vi "GageTransfer-LowOverheadMod.vi"(0 "Handle Cluster":T1, 1 "Start (0)":dbl, 2 "Length (4096)":dbl=4096.0, 5 "Buffer in I32":i32[](array[numeric]), 7 "Buffer in I16":i16[](array[numeric]), 9 "Buffer in U8":u8[](array[numeric]), 12 "Channel (0)":u16 step=1, 13 "Mode (0)":u32 step=1, 14 "Segment (1)":u32=1) -> (3 "Actual Length":dbl, 4 "Actual Start":dbl, 6 "Buffer Out I32":i32[](array[numeric]), 8 "Buffer Out I16":i16[](array[numeric]), 10 "Buffer Out U8":u8[](array[numeric]), 15 "Error Code":i32)   [LabVIEW 2014, in "GageLv.lvlib"]
doc: "This VI transfers the data from one channel of the CompuScope system identified by Handle Cluster, which is obtained by calling CsTool-GetSystem.vi. For accurate interpretation of the transferred data, the user should always use the returned Actual Start and Actual Length, and not the requested values. \n\nThis VI can be used for transferring data from 8, 12, 14, and 16 bit CompuScope hardware. Data are transferred from on-board CompuScope memory to PC RAM using PCI Bus Mastering at rates of up to 200 MB/s. \n\nInternally, CsTool-Transfer.vi converts the raw integer ADC code values into double variable voltage values. For more rapid data access, the user may remove the voltage conversion step. The VI will not return programmatic control to LabVIEW until all of the data have been transferred. \n\nIf the call is successful, a 1 is returned in the Error Code indicator. If the call is unsuccessful, an appropriate error code is returned. A descriptive error string may be obtained by calling CsTool-ErrorHandler.vi.\n\n\nInput Value Descriptions:\n\nChannel\nThis integer value specifies the channel from which data are to be transferred. The default value is 0 for the first channel in the CompuScope system. Channels in a LabVIEW CompuScope system begin at 0. If an invalid channel number is given, an error will be returned. Please see the CompuScope hardware manual for more information on channel enumeration.\n\nMode\nThis integer value determines the current transfer mode. Currently, the only valid value for this input is 0.\n\nSegment(1)\nThis integer value determines which Multiple Record segment is to be transferred, if the CompuScope hardware was operating in Multiple Record Mode. For Single Record Mode acquisitions, the user must always set the Record value to 1, which is the default value. If the Record value is too large, an error code will be returned. \n\nStart\nThis double variable value determines the requested starting point of the data transfer from CompuScope memory to PC RAM. Start is specified relative to the trigger address for the acquisition. A Start value of 0 will cause data transfer to begin at the trigger address. Negative Start values are used for the transfer of pre-trigger data. Positive Start values may be used to begin transfer after the trigger address. The default Start value is 0. \n\nLength\nThis double variable value specifies the amount of data, in samples, to be transferred. The default value is 4096. \n\nData in Volts\nThis array variable, of type double, is the LabVIEW buffer variable into which transferred data are returned. The size of the array will be at least Length samples. Data are returned as voltage values, whose conversion depends upon the resolution of the CompuScope system and on the current input range.\n\nActual Start\nThis double variable value returns the actual start point of the data array. The Actual Start may be lower than the requested Start value. This is because the CompuScope memory architecture may force the drivers to download data from an earlier point than the start position. For example, if Start is input to CsTool-Transfer.vi as 0, the Actual Start may return as -2, indicating that two extra samples were returned before the Start position. \n\nThe user must account for the discrepancy between the Start and the Actual Start. The user may choose to ignore samples transferred from before the Start position. Alternatively, the user may conserve these samples, accounting for the fact that the values begin at Actual Start. \n\nActual Length\nThis double variable value returns the actual amount of data transferred, which may be different from the requested Length. The difference, if any, results from CompuScope memory architecture."
uses:
  <instrlib>/GageLv_uic/GageLv.lvlib
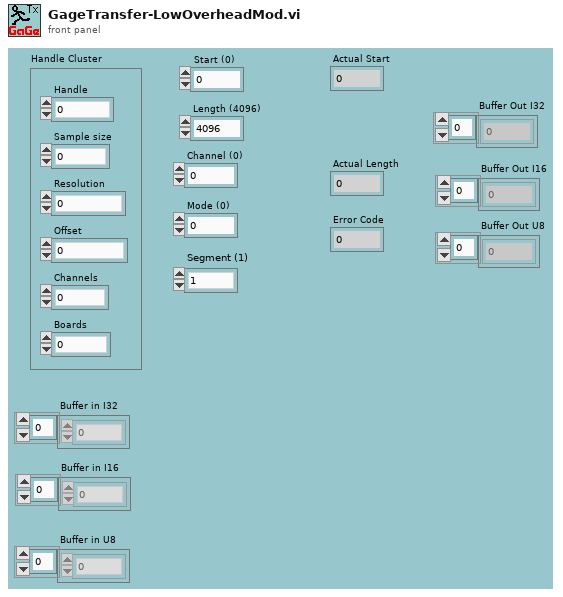
[diagram p1: front panel]
types:
  T1 = cluster{"Handle":u32, "Sample size":u32, "Resolution":i32, "Offset":i32, "Channels":u32, "Boards":u32}
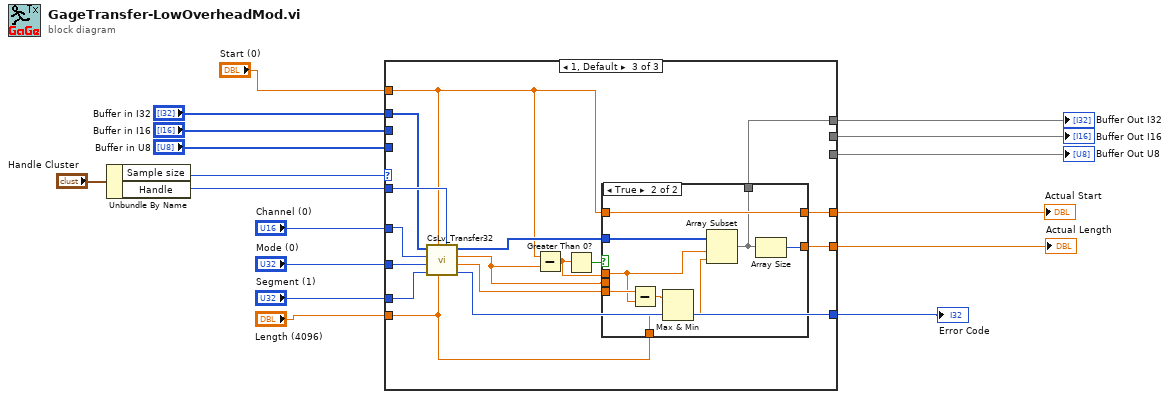
[diagram p0: block diagram]
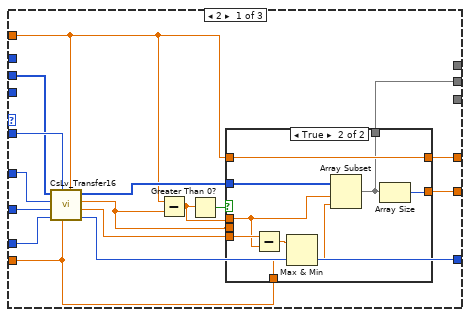
[diagram p2: hidden frame]
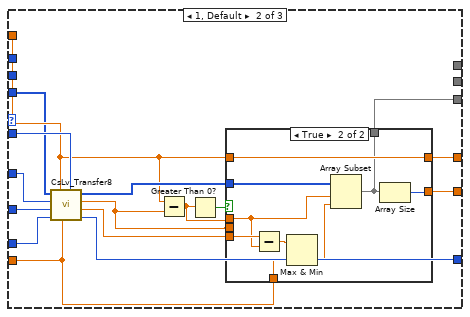
[diagram p4: hidden frame]
diagram:
  n1 = Unbundle By Name("Handle Cluster") -> ("Sample size"=w17:u32, "Handle"=w16:u32)
  n2 = case shown="1, Default" w17 {
    tunnel: "Length (4096)" -> [w24 w52 w80]
    tunnel: "Segment (1)" -> [w31 w59 w87]
    tunnel: "Mode (0)" -> [w30 w58 w86]
    tunnel: "Start (0)" -> [w23 w51 w79]
    tunnel: [w33 w61 w89] -> w13
    tunnel: w16 -> [w32 w60 w88]
    tunnel: "Channel (0)" -> [w29 w57 w85]
    tunnel: "Buffer in U8" -> [_ w48 _]
    tunnel: "Buffer in I16" -> [w18 _ _]
    tunnel: "Buffer in I32" -> [_ _ w74]
    tunnel: [w22 w50 w78] -> w6
    tunnel: [w21 w49 w77] -> w5
    tunnel: [w20 _ _] -> w4
    tunnel: [_ w47 _] -> w2
    tunnel: [_ _ w76] -> w1
    frame 2 {
      n3 = call <instrlib>:"CsLv_Transfer16.vi"("Start (0)"=w23, "Length (4096)"=w24, "Handle"=w32, "Segment (1)"=w31, "Mode (0)"=w30, "Channel (0)"=w29, "Buffer in I16"=w18) -> ("Error Code"=w33:i32, "Actual Length"=w25:dbl, "Actual Start"=w19:dbl, "Buffer"=w26:i16[])  [unwired: 1 in]
      n4 = Subtract(x=w23, y=w19) -> (x-y=w28:dbl)
      n5 = Greater Than 0?(x=w28) -> (x > 0?=w27:bool)
      n6 = case shown="True" w27 {
        tunnel: w28 -> [_ w43]
        tunnel: w25 -> [w36 w44]
        tunnel: [w36 w45] -> w22
        tunnel: w24 -> [_ w40]
        tunnel: w26 -> [w34 w39]
        tunnel: [w35 w38] -> w21
        tunnel: w23 -> [_ w38]
        tunnel: w19 -> [w35 _]
        tunnel: [w34 w37] -> w20
        frame False {
        }
        frame True {
          n7 = Subtract(x=w44, y=w43) -> (x-y=w42:dbl)
          n8 = Max & Min(x=w42, y=w40) -> (min(x,y)=w41:dbl)  [unwired: 1 out]
          n9 = Array Subset(array=w39, index=w43, length=w41) -> (w37:i16[])
          n10 = Array Size(array=w37) -> (size(s)=w45:i32)
        }
      }
    }
    frame 1, Default {
      n11 = call <instrlib>:"CsLv_Transfer8.vi"("Handle"=w60, "Length (4096)"=w52, "Start (0)"=w51, "Segment (1)"=w59, "Mode (0)"=w58, "Channel (0)"=w57, "Buffer in"=w48) -> ("Error Code"=w61:i32, "Actual Length"=w53:dbl, "Actual Start"=w46:dbl, "Buffer out"=w54:u8[])  [unwired: 1 in]
      n12 = Subtract(x=w51, y=w46) -> (x-y=w56:dbl)
      n13 = Greater Than 0?(x=w56) -> (x > 0?=w55:bool)
      n14 = case shown="True" w55 {
        tunnel: w56 -> [_ w71]
        tunnel: w53 -> [w64 w72]
        tunnel: [w64 w73] -> w50
        tunnel: w52 -> [_ w68]
        tunnel: w54 -> [w62 w67]
        tunnel: [w63 w66] -> w49
        tunnel: w51 -> [_ w66]
        tunnel: w46 -> [w63 _]
        tunnel: [w62 w65] -> w47
        frame False {
        }
        frame True {
          n15 = Subtract(x=w72, y=w71) -> (x-y=w70:dbl)
          n16 = Max & Min(x=w70, y=w68) -> (min(x,y)=w69:dbl)  [unwired: 1 out]
          n17 = Array Subset(array=w67, index=w71, length=w69) -> (w65:u8[])
          n18 = Array Size(array=w65) -> (size(s)=w73:i32)
        }
      }
    }
    frame 4 {
      n19 = call <instrlib>:"CsLv_Transfer32.vi"("Handle"=w88, "Length (4096)"=w80, "Start (0)"=w79, "Segment (1)"=w87, "Mode (16)"=w86, "Channel (0)"=w85, "Buffer in"=w74) -> ("Error Code"=w89:i32, "Actual Length"=w81:dbl, "Actual Start"=w75:dbl, "Buffer out"=w82:i32[])  [unwired: 1 in]
      n20 = Subtract(x=w79, y=w75) -> (x-y=w84:dbl)
      n21 = Greater Than 0?(x=w84) -> (x > 0?=w83:bool)
      n22 = case shown="True" w83 {
        tunnel: w84 -> [_ w99]
        tunnel: w81 -> [w92 w100]
        tunnel: [w92 w101] -> w78
        tunnel: w80 -> [_ w96]
        tunnel: w82 -> [w90 w95]
        tunnel: [w91 w94] -> w77
        tunnel: w79 -> [_ w94]
        tunnel: w75 -> [w91 _]
        tunnel: [w90 w93] -> w76
        frame False {
        }
        frame True {
          n23 = Subtract(x=w100, y=w99) -> (x-y=w98:dbl)
          n24 = Max & Min(x=w98, y=w96) -> (min(x,y)=w97:dbl)  [unwired: 1 out]
          n25 = Array Subset(array=w95, index=w99, length=w97) -> (w93:i32[])
          n26 = Array Size(array=w93) -> (size(s)=w101:i32)
        }
      }
    }
  }
  "Buffer Out U8" <- w2
  "Actual Length" <- w6
  "Error Code" <- w13
  "Actual Start" <- w5
  "Buffer Out I16" <- w4
  "Buffer Out I32" <- w1
